vi "Update Focus.vi"(8 "error in (no error)":errorcluster, 10 "Focus region centers":dbl[](array[numeric]), 11 "Spectrum Recorder too in":refnum<class "Spectrum Recorder too.lvclass">) -> (0 "error out":errorcluster, 3 "Spectrum Recorder too out":refnum<class "Spectrum Recorder too.lvclass">)   [LabVIEW 2016, in "Spectrum Recorder too.lvclass"]
uses:
  Spectrum Recorder too.lvclass
  NHMFL_Core/Libraries/Red Pitaya/RP Core/Red Pitaya Transceiver Driver/Spectrum Configuration.ctl
  Spectrum Recorder too.lvclass/Spectrum Recorder too.ctl
  Write Spectrum Recorder Configuration.vi
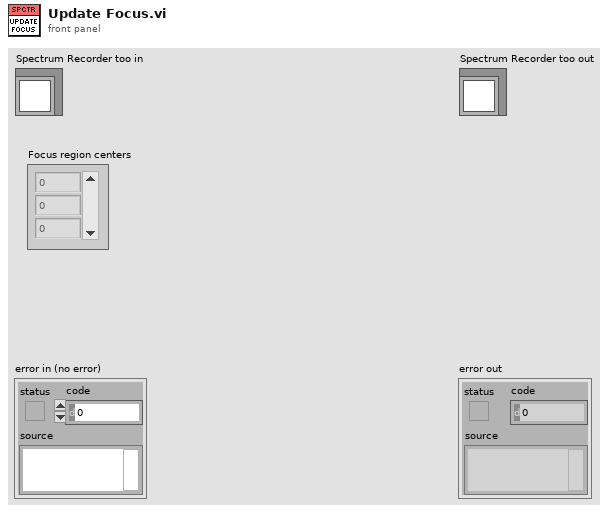
[diagram p1: front panel]
types:
  T1 = typedef "Spectrum Configuration.ctl" = cluster{"Start frequency":dbl, "End frequency":dbl, "Coarse step":dbl, "Step duration":dbl, "Red Pitaya address":string, "Open plot \non start":bool, "Fine region centers":dbl[], "Regions width":dbl, "Fine step":dbl, "Pause between scans":dbl, "Clear rgs on start":bool, "Output amplitude":dbl}
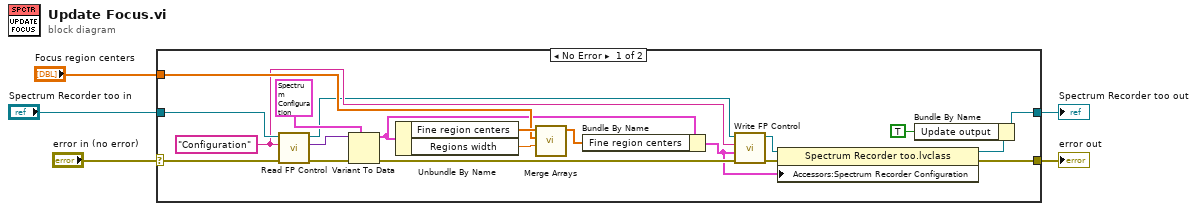
[diagram p0: block diagram]
diagram:
  n1 = case shown="No Error" "error in (no error)" {
    selector: "error in (no error)" -> [w13 w27]
    tunnel: [w8 w27] -> w4
    tunnel: [w7 w26] -> w2
    tunnel: "Spectrum Recorder too in" -> [w19 w26]
    tunnel: "Focus region centers" -> [w20 _]
    frame No Error {
      w16 = "Configuration" ("Control Name")
      n2 = call-dynamic "Read FP Control.vi"("error in (no error)"=w13, "Control Name"=w16, "Measure Object in"=w19) -> ("error out"=w25:errorcluster, "Control Value"=w24:variant, "Measure Object out"=w14:refnum<class "Spectrum Recorder too.lvclass">)  [unwired: 5 in, 1 out]
      n3 = Variant To Data(error in=w25, type=T1 {"Start frequency"=500000.0, "End frequency"=2000000.0, "Coarse step"=40.0, "Step duration"=0.004, "Red Pitaya address"="192.168.1.100", "Open plot \non start"=TRUE, "Fine region centers"=[], "Regions width"=2000.0, "Fine step"=20.0, "Pause between scans"=0.0, "Clear rgs on start"=FALSE, "Output amplitude"=1.0} ("Configuration"), Variant=w24) -> (data=w18:T1, error out=w15:errorcluster)
      n4 = Unbundle By Name(w18) -> ("Fine region centers"=w22:dbl[], "Regions width"=w21:dbl)
      n5 = call "Merge Arrays.vi"("Coerce window width"=w21, "New Array"=w20, "Old Array"=w22) -> ("New Array out"=w17:dbl[])  [unwired: 8 in]
      n6 = Bundle By Name(cluster=w18, "Fine region centers"=w17) -> (w10:T1)
      n7 = call-dynamic "Write FP Control.vi"("error in (no error)"=w15, "Control Value"=w10, "Control Name"=w16, "Measure Object in"=w14) -> ("error out"=w12:errorcluster, "Measure Object out"=w11:refnum<class "Spectrum Recorder too.lvclass">)  [unwired: 6 in]
      n8 = property class="Spectrum Recorder too.lvclass"(reference=w11, error in=w12, "Accessors:Spectrum Recorder Configuration"=w10) -> (reference out=w9:refnum<class "Spectrum Recorder too.lvclass">, error out=w8:errorcluster)
      n9 = Bundle By Name(cluster=w9, "Update output"=TRUE) -> (w7:refnum<class "Spectrum Recorder too.lvclass">)
    }
    frame Error {
    }
  }
  "error out" <- w4
  "Spectrum Recorder too out" <- w2
